vi "Sequence.BuildNewRow.vi"(10 "Syntax":string, 11 "UI.Sequence#ofColumns":i32) -> (3 "New Array":string[](array[string]))   [LabVIEW 2015, in "Simple Sequence Tools - Editor.lvlib"]
uses:
  Simple Sequence Tools - Editor.lvlib
  Shared/SubVIs/Main.Constants.vi
  Shared/Simple Sequence Tools - Shared.lvlib
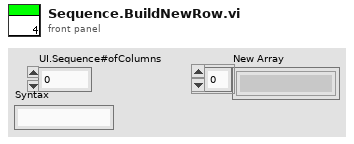
[diagram p1: front panel]
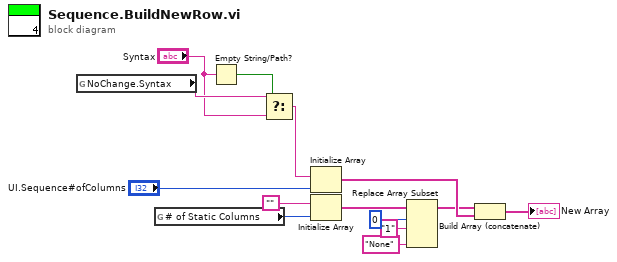
[diagram p0: block diagram]
diagram:
  n1 = global read "Main.Constants.vi" "NoChange.Syntax"() -> (w3:string)
  n2 = global read "Main.Constants.vi" "# of Static Columns"() -> (w9:u32)
  n3 = Empty String/Path?(string/path="Syntax") -> (empty?=w4:bool)
  n4 = Select(t=w3, s=w4, f="Syntax") -> (s? t:f=w2:string)
  n5 = Initialize Array(w2, "UI.Sequence#ofColumns") -> (w12:string[])
  n6 = Initialize Array("", w9) -> (w11:string[])
  n7 = Replace Array Subset(array=w11, new element #1="1" ("new element/subarray"), index #1=0 ("index"), new element #2="None" ("new element/subarray")) -> (w8:string[])  [unwired: 1 in]
  n8 = Build Array (concatenate)(w8, w12) -> (→"New Array":string[])
